vi "Config.vi"(8 "error in (no error)":errorcluster, 10 "Setting_Config":variant, 11 "Keysight 5700C in":refnum<class "Keysight 5700C.lvclass">) -> (0 "error out":errorcluster, 3 "Keysight 5700C out":refnum<class "Keysight 5700C.lvclass">)   [LabVIEW 2019, in "Concrete.lvlib" / "Keysight 5700C.lvclass"]
uses:
  Keysight 5700C.lvclass
  Keysight 5700C.lvclass/Keysight 5700C.ctl
panel:
  in  "Setting":T1={"Max. Volt"=10.0, "Current Limit"=0.5, "Volt Level"=10.0}
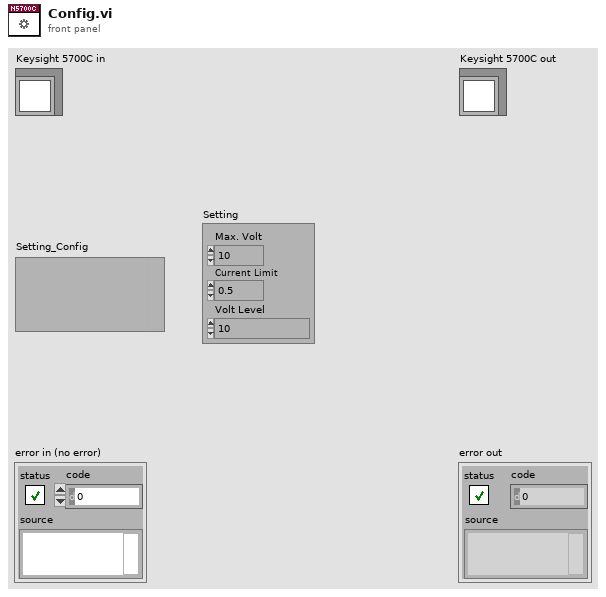
[diagram p1: front panel]
types:
  T1 = cluster{"Max. Volt":dbl, "Current Limit":dbl, "Volt Level":dbl}
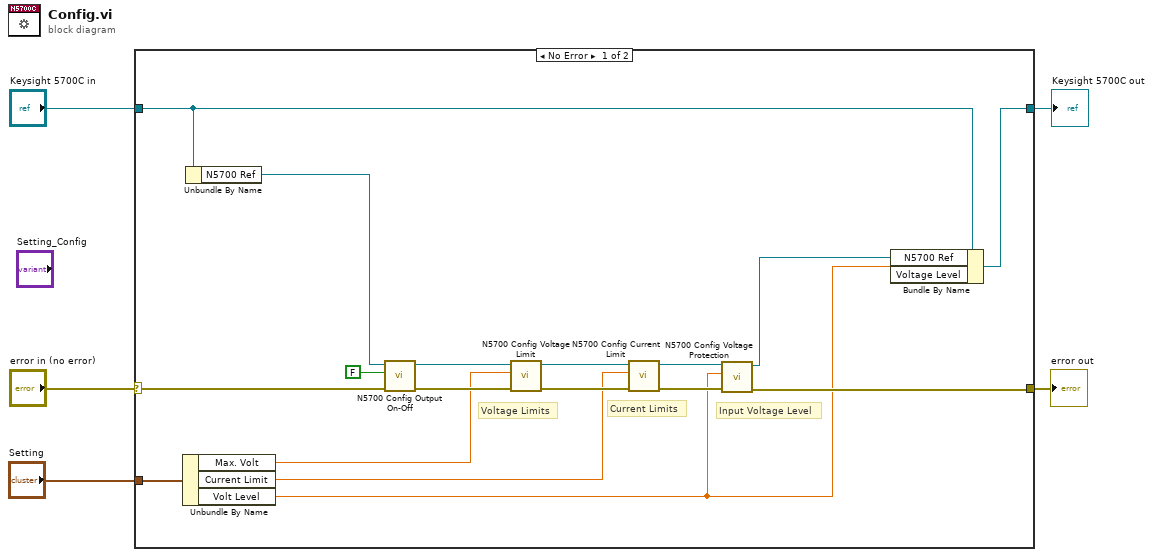
[diagram p0: block diagram]
diagram:
  n1 = case shown="No Error" "error in (no error)" {
    selector: "error in (no error)" -> [w15 w24]
    tunnel: [w9 w24] -> w4
    tunnel: [w22 w23] -> w2
    tunnel: "Keysight 5700C in" -> [w14 w23]
    tunnel: "Setting" -> [w16 _]
    frame No Error {
      # "Input Voltage Level"
      # "Current Limits"
      # "Voltage Limits"
      n2 = Unbundle By Name(w16) -> ("Max. Volt"=w19:dbl, "Current Limit"=w12:dbl, "Volt Level"=w8:dbl)
      n3 = Unbundle By Name(w14) -> ("N5700 Ref"=w13:refnum<visa-resource-name>)
      n4 = call <instrlib>:"N5700 Config Output On-Off.vi"("error"=w15, "Output ON"=FALSE ("enabled (True)"), "VISA"=w13) -> ("error out"=w20:errorcluster, "VISA out"=w21:refnum<visa-resource-name>)  [unwired: 4 in]
      n5 = call <instrlib>:"N5700 Config Voltage Limit.vi"("error"=w20, "Volt Limit"=w19, "VISA"=w21) -> ("error out"=w17:errorcluster, "VISA out"=w18:refnum<visa-resource-name>)  [unwired: 4 in]
      n6 = call <instrlib>:"N5700 Config Current Limit.vi"("error"=w17, "Current Limit"=w12, "VISA"=w18) -> ("error out"=w11:errorcluster, "VISA out"=w10:refnum<visa-resource-name>)  [unwired: 4 in]
      n7 = call <instrlib>:"N5700 Config Voltage Protection.vi"("error"=w11, "OVP Level"=w8, "VISA"=w10) -> ("error out"=w9:errorcluster, "VISA out"=w6:refnum<visa-resource-name>)  [unwired: 4 in]
      n8 = Bundle By Name(cluster=w14, "N5700 Ref"=w6, "Voltage Level"=w8) -> (w22:refnum<class "Keysight 5700C.lvclass">)
    }
    frame Error {
    }
  }
  "error out" <- w4
  "Keysight 5700C out" <- w2
